vi "Write Generated files.vi"(8 "error in (no error)":errorcluster, 10 "Generated files":path[](array[path]), 11 "Build Named Build Specification Data in":refnum<class "Build Named Build Specification Data.lvclass">) -> (0 "error out":errorcluster, 3 "Build Named Build Specification Data out":refnum<class "Build Named Build Specification Data.lvclass">)   [LabVIEW 2020, in "ProjectBuilder.lvlib" / "Build Named Build Specification Data.lvclass"]
uses:
  Build Named Build Specification Data.lvclass
  Build Named Build Specification Data.lvclass/Build Named Build Specification Data.ctl
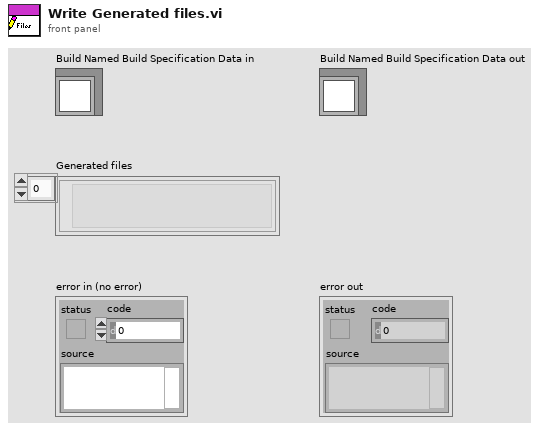
[diagram p1: front panel]
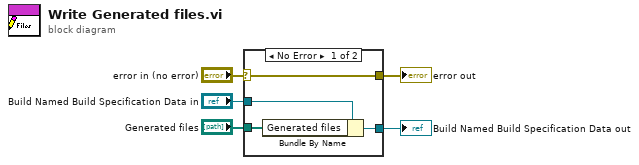
[diagram p0: block diagram]
diagram:
  n1 = case shown="No Error" "error in (no error)" {
    selector: "error in (no error)" -> [w9 w10]
    tunnel: [w9 w10] -> w4
    tunnel: [w7 w11] -> w2
    tunnel: "Build Named Build Specification Data in" -> [w8 w11]
    tunnel: "Generated files" -> [w6 _]
    frame No Error {
      n2 = Bundle By Name(cluster=w8, "Generated files"=w6) -> (w7:refnum<class "Build Named Build Specification Data.lvclass">)
    }
    frame Error {
    }
  }
  "error out" <- w4
  "Build Named Build Specification Data out" <- w2
